vi "showCursors.vi"(8 "error in (no error)":errorcluster, 10 "Coords":T1, 11 "QControl_Graph in":refnum<class "QControl_Graph.lvclass">) -> (0 "error out":errorcluster, 3 "QControl_Graph out":refnum<class "QControl_Graph.lvclass">)   [LabVIEW 2017, in "QControl_Graph.lvclass"]
uses:
  QControl_Graph.lvclass
  Applications/National Instruments/LabVIEW 2017 64-bit/vi.lib/QSI/QControls/QControl Classes/WaveformGraph/WaveformGraph.lvclass
  <vilib>/Utility/miscctls.llb/LVPoint32TypeDef.ctl
  QControl_Graph.lvclass/QControl_Graph.ctl
  Users/benji667/Downloads/Graph-Extensions-LabVIEW-master/LV2014/Graph Extensions.lvlib
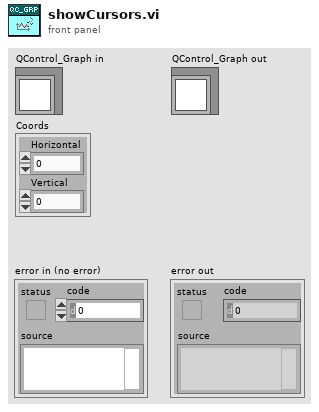
[diagram p1: front panel]
types:
  T1 = typedef "LVPoint32TypeDef.ctl" = cluster{"Horizontal":i32, "Vertical":i32}
  T2 = cluster{"font":cluster{"Font Name":string, "Size":i16, "Strikeout?":bool, "Italic?":bool, "Underline?":bool, "Outline?":bool, "Shadow?":bool, "Bold?":bool}, "size":i16, "Timestamp":enum16{"at TOP", "at BOTTOM", "none"}, "Vertical Line?":bool, "Horizontal Line?":bool, "alignment(left, top)":cluster{"horizontal":enum16{"left", "center", "right"}, "vertical":enum16{"top", "center", "bottom"}}, "TextFormat":string, "time format (%H:%M:%S)":string}
  T3 = typedef "QControl_Graph.lvclass/Cursor Properties.ctl" = cluster{"font":T4, "size":i16, "time format (%H:%M:%S)":string, "Vertical Line?":bool, "Horizontal Line?":bool, "alignment(left, top)":T5, "TextFormat":string, "Timestamp":enum16{"at TOP", "at BOTTOM", "none"}}
  T4 = typedef "QControl_Graph.lvclass/Font.ctl" = cluster{"Font Name":string, "Size":i16, "Strikeout?":bool, "Italic?":bool, "Underline?":bool, "Outline?":bool, "Shadow":bool, "Bold?":bool}
  T5 = typedef "QControl_Graph.lvclass/Alignment.ctl" = cluster{"Horizontal":T6, "Vertical":T7}
  T6 = typedef "QControl_Graph.lvclass/Alignment.Horizontal.ctl" = enum16{"left", "center", "right"}
  T7 = typedef "QControl_Graph.lvclass/Alignment.Vertical.ctl" = enum16{"top", "center", "bottom"}
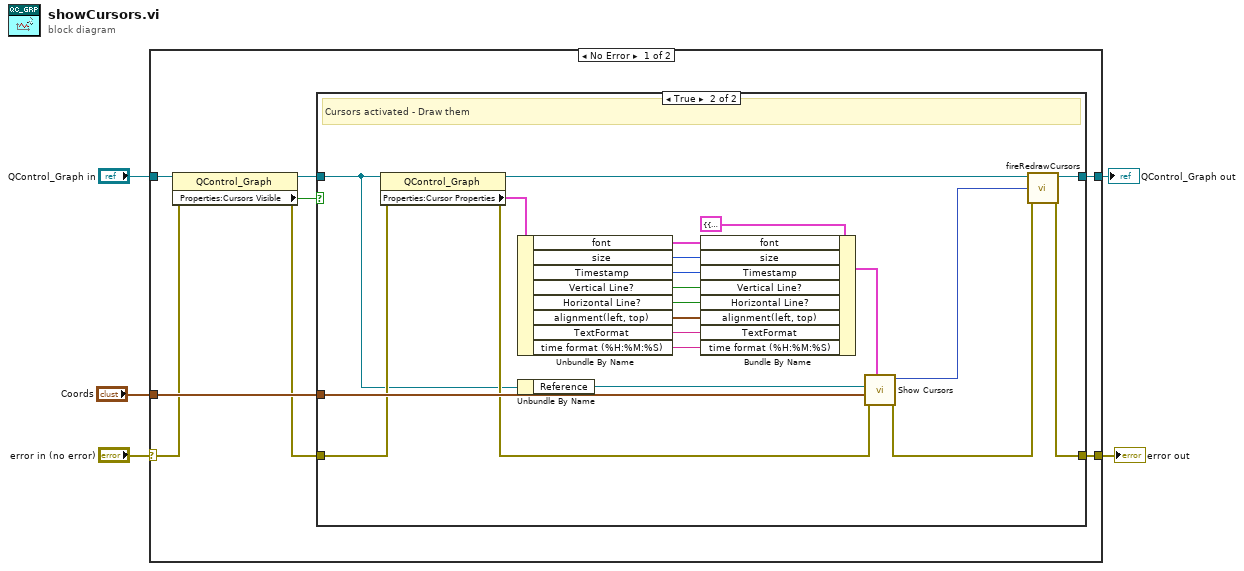
[diagram p0: block diagram]
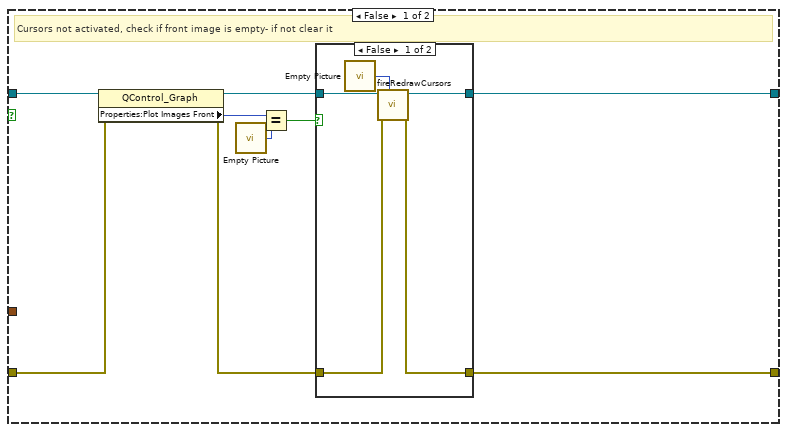
[diagram p2: hidden frame]
diagram:
  n1 = case shown="No Error" "error in (no error)" {
    selector: "error in (no error)" -> [w8 w52]
    tunnel: [w10 w52] -> w4
    tunnel: [w12 w51] -> w2
    tunnel: "QControl_Graph in" -> [w13 w51]
    tunnel: "Coords" -> [w11 _]
    frame No Error {
      n2 = property class="QControl_Graph"(reference=w13, error in=w8) -> (reference out=w9:refnum<class "QControl_Graph.lvclass">, error out=w7:errorcluster, "Properties:Cursors Visible"=w6:bool)
      n3 = case shown="True" w6 {
        tunnel: [w16 w32] -> w12
        tunnel: w11 -> [_ w50]
        tunnel: [w14 w30] -> w10
        tunnel: w9 -> [w22 w36]
        tunnel: w7 -> [w19 w38]
        frame False {
          # "Cursors not activated, check if front image is empty- if not clear it"
          n4 = property class="QControl_Graph"(reference=w22, error in=w19) -> (reference out=w17:refnum<class "QControl_Graph.lvclass">, error out=w15:errorcluster, "Properties:Plot Images Front"=w21:picture)
          n5 = call "Empty Picture"() -> ("empty picture"=w20:picture)
          n6 = Equal?(x=w21, y=w20) -> (x = y?=w18:bool)
          n7 = case shown="False" w18 {
            tunnel: w17 -> [w27 w29]
            tunnel: [w26 w29] -> w16
            tunnel: w15 -> [w25 w28]
            tunnel: [w24 w28] -> w14
            frame False {
              n8 = call "Empty Picture"() -> ("empty picture"=w23:picture)
              n9 = call-dynamic "fireRedrawCursors.vi"("Cursors"=w23, "error in (no error)"=w25, "QControl_Graph in"=w27) -> ("error out"=w24:errorcluster, "QControl_Graph out"=w26:refnum<class "QControl_Graph.lvclass">)  [unwired: 7 in]
            }
            frame True {
            }
          }
        }
        frame True {
          # "Cursors activated - Draw them"
          n10 = property class="QControl_Graph"(reference=w36, error in=w38) -> (reference out=w33:refnum<class "QControl_Graph.lvclass">, error out=w37:errorcluster, "Properties:Cursor Properties"=w47:T3)
          n11 = Unbundle By Name(w47) -> ("font"=w46:T4, "size"=w45:i16, "Timestamp"=w44:enum16{"at TOP", "at BOTTOM", "none"}, "Vertical Line?"=w43:bool, "Horizontal Line?"=w42:bool, "alignment(left, top)"=w41:T5, "TextFormat"=w40:string, "time format (%H:%M:%S)"=w39:string)
          n12 = Unbundle By Name(w36) -> ("Reference"=w35:refnum<vi>)
          n13 = Bundle By Name(cluster=T2 {"font"={"Font Name"="Arial", "Size"=14, "Strikeout?"=FALSE, "Italic?"=FALSE, "Underline?"=FALSE, "Outline?"=FALSE, "Shadow?"=FALSE, "Bold?"=FALSE}, "size"=1, "Timestamp"=enum."at TOP", "Vertical Line?"=FALSE, "Horizontal Line?"=FALSE, "alignment(left, top)"={"horizontal"=enum."center", "vertical"=enum."center"}, "TextFormat"="%2$.2f\\n\\n%1$s", "time format (%H:%M:%S)"="%H:%M%:S"} ("Cursor Options"), "font"=w46, "size"=w45, "Timestamp"=w44, "Vertical Line?"=w43, "Horizontal Line?"=w42, "alignment(left, top)"=w41, "TextFormat"=w40, "time format (%H:%M:%S)"=w39) -> (w48:T2)
          n14 = call "Show Cursors.vi"("Cursor Options"=w48, "error in (no error)"=w37, "Coords"=w50, "XY Graph"=w35) -> ("error out"=w31:errorcluster, "output picture"=w34:picture)  [unwired: 6 in]
          n15 = call-dynamic "fireRedrawCursors.vi"("Cursors"=w34, "error in (no error)"=w31, "QControl_Graph in"=w33) -> ("error out"=w30:errorcluster, "QControl_Graph out"=w32:refnum<class "QControl_Graph.lvclass">)  [unwired: 7 in]
        }
      }
    }
    frame Error {
    }
  }
  "error out" <- w4
  "QControl_Graph out" <- w2
